vi "Test Get Summary of Case Not Executed.vi"(8 "error in (no error)":errorcluster, 11 "Result Model Result Recording Test in":refnum<class "Result Model Result Recording Test.lvclass">) -> (0 "error out":errorcluster, 3 "Result Model Result Recording Test out":refnum<class "Result Model Result Recording Test.lvclass">)   [LabVIEW 2020, in "Result Model Result Recording Test.lvclass"]
uses:
  Result Model Result Recording Test.lvclass
  ae2c71b8-32bb-49d1-8500-0119bfec74ff.vi
  source/User Interface/Result Model/Result Model.lvclass
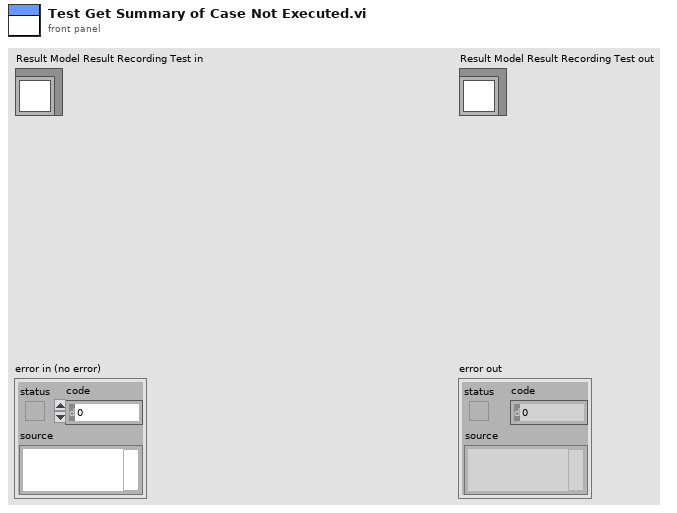
[diagram p1: front panel]
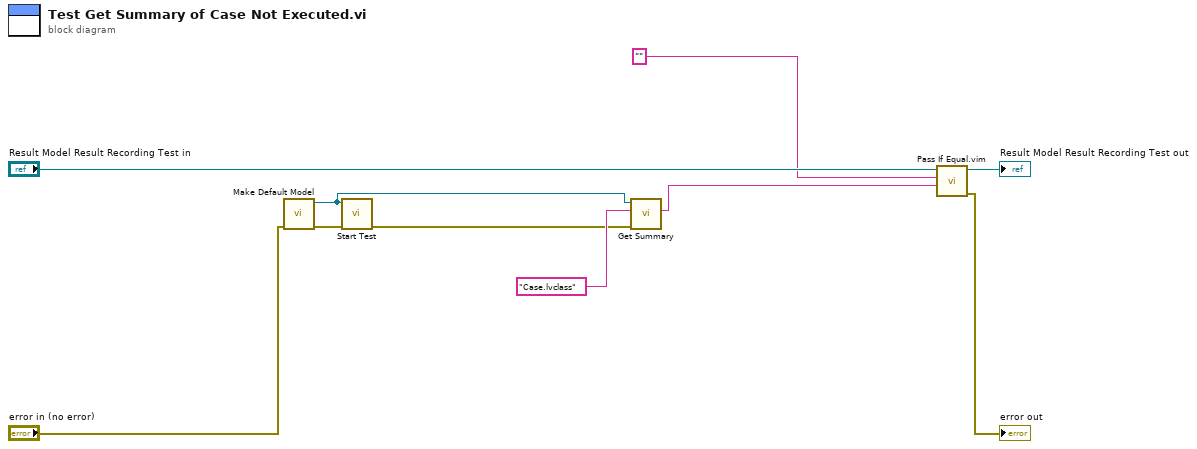
[diagram p0: block diagram]
diagram:
  n1 = call "Make Default Model.vi"("error in (no error)"="error in (no error)") -> ("error out"=w3:errorcluster, "Result Model out"=w1:refnum<class "Result Model.lvclass">)  [unwired: 9 in]
  n2 = call "Start Test.vi"("error in (no error)"=w3, "Result Model by Reference In"=w1) -> ("error out"=w2:errorcluster)  [unwired: 9 in]
  n3 = call "Get Summary.vi"("error in (no error)"=w2, "Item"="Case.lvclass", "Result Model by Reference In"=w1) -> ("Summary"=w4:string)  [unwired: 7 in, 1 out]
  n4 = call "Pass If Equal.vim"("Actual"=w4, "Expected"="", "LUnit Test Case In"="Result Model Result Recording Test in") -> ("error out"=→"error out":errorcluster, "LUnit Test Case Out"=→"Result Model Result Recording Test out":refnum<class "Result Model Result Recording Test.lvclass">)  [unwired: 7 in]
